vi "E725_Sample_Application_1.vi"() -> ()   [LabVIEW 2009]
doc: "This VI demonstrates how to initialize an E-712 system, how to move one connected axis and how to query for the position value of this axis. \n\nIn this example the E-712 is connected through COM port 1 with baudrate 115200. The VI runs E712_Configuration_Setup.vi with these specified settings, moves the first connected axis relative to its current position and reads the position of this axis. The diagram shows how to combine the driver VIs for these tasks. \n\nWarning: Before running this VI, modify the \"Interface\" and \"RS232 settings\" (or \"TCP/IP settings\" or \"USB settings\") to reflect your configuration. The predefined settings provided with the VI probably do not match your system."
panel:
  in  "stop":bool
  in  "error in":errorcluster
  out "Running":bool caption="Configuration_Setup.vi is running"
  out "error out":errorcluster
  out "Position":dbl[](array[numeric]) format="%.6f"
  out "Conn. Axis":string[](array[string])
  out "Identification":string
  # "This VI demonstrates how to initialize an E-712 system, how to move one axis and how to query for the position value of this axis. \nThe VI runs E712_Configuration_Setup.vi with specified settings, moves the first axis relative to its current position and reads the\nposition of this axis. The diagram shows how to combine the driver VIs for these tasks. \n\nWarning: Before running this VI, modify the interface settings on the block diagram to reflect your configuration. The predefined \n                 settings provided with the VI probably do not match your system."
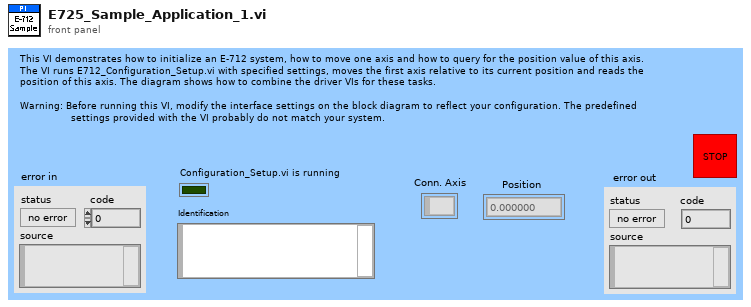
[diagram p1: front panel]
types:
  T1 = cluster{"Host address/name":string, "Port":i32, "Board":i32, "TCP/IP Search?":bool}
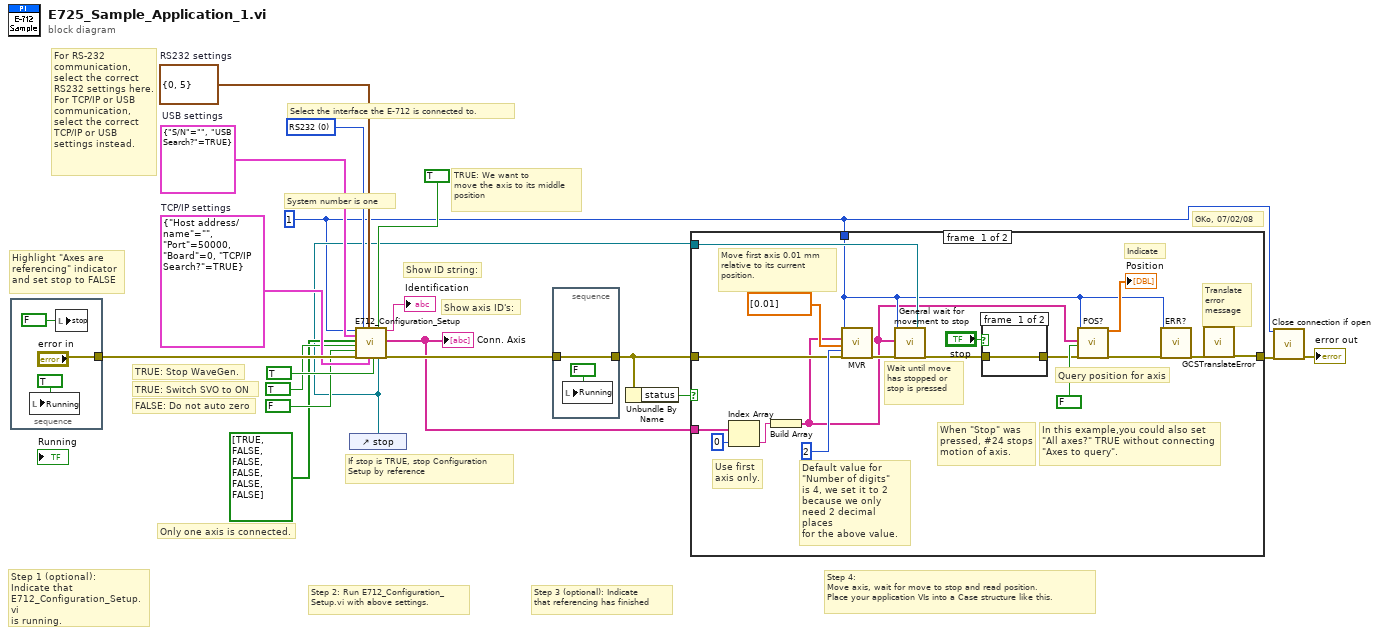
[diagram p0: block diagram]
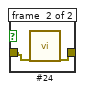
[diagram p2: hidden frame]
diagram:
  w5 = cluster{"S/N":string, "USB Search?":bool} {"S/N"="", "USB Search?"=TRUE}  # USB settings
  w6 = u16 0 items=["RS232", "TCP/IP", "USB"] ("Interface")
  w8 = cluster{"Portnumber":i32, "Baudrate":u16} {"Portnumber"=0, "Baudrate"=5}  # RS232 settings
  w14 = T1 {"Host address/name"="", "Port"=50000, "Board"=0, "TCP/IP Search?"=TRUE}  # TCP/IP settings
  w1 = 1 ("System no.")
  # "Only one axis is connected."
  # "TRUE: We want to\nmove the axis to its middle\nposition"
  # "FALSE: Do not auto zero"
  # "TRUE: Switch SVO to ON"
  # "If stop is TRUE, stop Configuration\nSetup by reference"
  # "Step 4: \nMove axis, wait for move to stop and read position.\nPlace your application VIs into a Case structure like this."
  # "For RS-232 \ncommunication,\nselect the correct\nRS232 settings here.\nFor TCP/IP or USB \ncommunication, \nselect the correct \nTCP/IP or USB\nsettings instead."
  # "Select the interface the E-712 is connected to."
  # "GKo, 07/02/08"
  # "Step 3 (optional): Indicate\nthat referencing has finished"
  # "Step 2: Run E712_Configuration_\nSetup.vi with above settings."
  # "Step 1 (optional): \nIndicate that\nE712_Configuration_Setup.vi\nis running."
  # "Highlight \"Axes are\nreferencing\" indicator\nand set stop to FALSE"
  # "Show axis ID's:"
  # "Show ID string:"
  # "TRUE: Stop WaveGen."
  # "System number is one"
  n1 = stacked-sequence {
    tunnel: ["error in"] -> w17
    frame #0 {
      n2 = local write "Running"(TRUE ("Running")) -> ()
      n3 = local write "stop"(FALSE ("stop")) -> ()
    }
  }
  n4 = control-ref of="stop"() -> (w4:refnum<vi>)
  n5 = call "E712_Configuration_Setup.vi"("System no."=w1, "USB settings"=w5, "Are stages connected?"=bool[] [TRUE, FALSE, FALSE, FALSE, FALSE, FALSE], "Change servo status to ON?"=TRUE ("Use dialog to define\nconnected stages?"), "Perform autozero?"=FALSE ("Use dialog to define\nconnected stages?"), "error in"=w17, "Interface"=w6, "RS232 settings"=w8, "TCP/IP settings"=w14, "Stop wave generator\noutput (if any)"=TRUE ("All axes?"), "Move to middle?"=TRUE, "Stop refnum"=w4) -> ("Identification"=→"Identification":string, "All conn. axes"=w13:string[], "error out"=w18:errorcluster)  [unwired: 3 in, 2 out]
  "Conn. Axis" <- w13
  n6 = stacked-sequence {
    tunnel: w18 -> [w24]
    tunnel: [w24] -> w16
    frame #0 {
      n7 = local write "Running"(FALSE ("Running")) -> ()
    }
  }
  n8 = Unbundle By Name(w16) -> ("status"=w15:bool)
  n9 = case shown="False" w15 {
    tunnel: [w36 w46] -> w2
    tunnel: w13 -> [w26 _]
    tunnel: w1 -> [w29 _]
    tunnel: w16 -> [w38 w46]
    tunnel: w4 -> [w35 _]
    frame #0 {
      # "Use first\naxis only."
      # "When \"Stop\" was \npressed, #24 stops\nmotion of axis."
      # "Translate\nerror \nmessage"
      # "Wait until move\nhas stopped or\nstop is pressed"
      # "Indicate"
      # "Default value for\n\"Number of digits\"\nis 4, we set it to 2\nbecause we only\nneed 2 decimal places\nfor the above value."
      # "Move first axis 0.01 mm\nrelative to its current\nposition."
      # "In this example,you could also set \n\"All axes?\" TRUE without connecting\n\"Axes to query\"."
      # "Query position for axis"
      n10 = Index Array(array=w26, index=0) -> (element=w27:string)
      n11 = Build Array(w27) -> (w25:string[])
      n12 = call "MVR.vi"("System no."=w29, "Axes to move"=w25, "Position values"=dbl[] [0.01], "No.of digits"=i16 2, "error in"=w38) -> ("error out"=w37:errorcluster)  [unwired: 14 in]
      n13 = call "General wait for movement to stop.vi"("System no."=w29, "Axes to wait for"=w25, "error in"=w37, "Stop refnum"=w35) -> ("error out"=w34:errorcluster)  [unwired: 14 in, 1 out]
      n14 = case shown="True" "stop" {
        tunnel: w34 -> [w43 w45]
        tunnel: [w43 w44] -> w33
        frame #0 {
        }
        frame #1 {
          n15 = call "#24.vi"("error in"=w45) -> ("error out"=w44:errorcluster)  [unwired: 18 in]
        }
      }
      n16 = call "POS?.vi"("System no."=w29, "Axes to query"=w25, "All axes?"=FALSE, "error in"=w33) -> ("Position"=→"Position":dbl[], "error out"=w31:errorcluster)  [unwired: 14 in]
      n17 = call "ERR?.vi"("System no."=w29, "error in"=w31) -> ("error out"=w30:errorcluster)  [unwired: 16 in, 1 out]
      n18 = call "GCSTranslateError.vi"("error in"=w30) -> ("error out"=w36:errorcluster)  [unwired: 16 in, 2 out]
    }
    frame #1 {
      # "Error during initialization"
    }
  }
  n19 = call "Close connection if open.vi"("System no."=w1, "error in"=w2) -> ("error out"=→"error out":errorcluster)  [unwired: 16 in, 1 out]
